vi "Begin.vi"(8 "error in":errorcluster) -> (0 "error out":errorcluster)   [LabVIEW 2014]
doc: "Called before other user functions, this VI is expected to open initial I/O refnums, load in file data, and do all program initialization. Notice that the <B>error out</B> terminal is simply used for data flow. Wiring it to other structures or subVIs ensures that this VI runs first."
uses:
  <vilib>/Rock Robotics/WPI/DriverStation/WPI_DriverStationRobotMode2.ctl
  <vilib>/Rock Robotics/WPI/Joystick/WPI_JoystickDeviceEnum.ctl
  <vilib>/Rock Robotics/WPI/Solenoid/WPI_SolenoidChannel.ctl
  <vilib>/Rock Robotics/SystemInterfaces/Typedef/FPGA_TypedefAnalogModuleForGyro.ctl
  <vilib>/Rock Robotics/SystemInterfaces/AI/FPGA_AIGyroChannel.ctl
  <vilib>/Rock Robotics/SystemInterfaces/AI/FPGA_AIChannel.ctl
  <vilib>/Rock Robotics/SystemInterfaces/Typedef/FPGA_TypedefAnalogModule.ctl
  <vilib>/Rock Robotics/WPI/Accelerometer/WPI_AccelerometerRange.ctl
  <vilib>/Rock Robotics/SystemInterfaces/DIO/FPGA_DIOChannel.ctl
  <vilib>/Rock Robotics/SystemInterfaces/Typedef/FPGA_TypedefDigitalModule.ctl
  <vilib>/Rock Robotics/WPI/CAN/TalonSRX/WPI_CANTalonSRX_APIControlMode.ctl
  Robot Global Data.vi
  <vilib>/Rock Robotics/WPI/Solenoid/WPI_SolenoidOpenSingle.vi
  <vilib>/Rock Robotics/WPI/Counter/WPI_CounterDigitalInputToDigitalSource.vi
  <vilib>/Rock Robotics/WPI/Accelerometer/InternalAccelerometer/WPI_AccelerometerInternalOpen.vi
  <vilib>/Rock Robotics/WPI/Switch/WPI_SwitchOpenLimit.vi
  <vilib>/Rock Robotics/WPI/RobotDrive/WPI_RobotDriveOpen4MotorWithCANTalonSRX.vi
  <vilib>/Rock Robotics/WPI/MotorControl/WPI_MotorControlOpenCANTalonSRX.vi
  <vilib>/Rock Robotics/WPI/Ultrasonic/WPI_SonarSRF04DigitalOpen.vi
  <vilib>/Rock Robotics/WPI/Ultrasonic/WPI_SonarSRF04DigitalRefNum Registry Set.vi
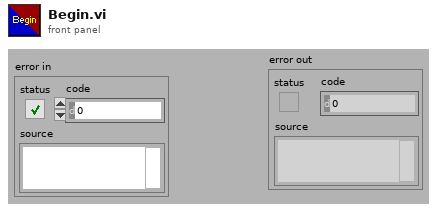
[diagram p1: front panel]
types:
  T1 = typedef "FPGA_DIOChannel.ctl" = enum8{"DIO 0", "DIO 1", "DIO 2", "DIO 3", "DIO 4", "DIO 5", "DIO 6", "DIO 7", "DIO 8", "DIO 9", "DIO MXP 0", "DIO MXP 1", "DIO MXP 2", "DIO MXP 3", "DIO MXP 4", "DIO MXP 5", "DIO MXP 6", "DIO MXP 7", "DIO MXP 8", "DIO MXP 9", "DIO MXP 10", "DIO MXP 11", "DIO MXP 12", "DIO MXP 13", "DIO MXP 14", "DIO MXP 15", "Invalid"}
  T2 = typedef "FPGA_TypedefDigitalModule.ctl" = enum16{"Controller 1"}
  T3 = typedef "WPI_CANTalonSRX_APIControlMode.ctl" = enum8{"Percent VBus", "Speed", "Position", "Slave", "Unchanged / Invalid"}
  T4 = typedef "WPI_AccelerometerRange.ctl" = enum16{"+/- 2 g", "+/- 4 g", "+/- 8 g"}
  T5 = typedef "FPGA_TypedefAnalogModule.ctl" = enum16{"Controller 1"}
  T6 = typedef "FPGA_AIChannel.ctl" = enum8{"AI 0", "AI 1", "AI 2", "AI 3", "AI MXP 0", "AI MXP 1", "AI MXP 2", "AI MXP 3", "Invalid"}
  T7 = typedef "FPGA_AIGyroChannel.ctl" = enum8{"AI 0", "AI 1", "Invalid"}
  T8 = typedef "FPGA_TypedefAnalogModuleForGyro.ctl" = enum16{"Controller 1"}
  T9 = typedef "WPI_SolenoidChannel.ctl" = enum8{"Solenoid 0", "Solenoid 1", "Solenoid 2", "Solenoid 3", "Solenoid 4", "Solenoid 5", "Solenoid 6", "Solenoid 7", "Invalid"}
  T10 = typedef "WPI_JoystickDeviceEnum.ctl" = enum16{"USB 0", "USB 1", "USB 2", "USB 3", "USB 4", "USB 5"}
  T11 = typedef "WPI_DriverStationRobotMode2.ctl" = enum16{"Autonomous Disabled", "Autonomous Enabled", "Teleop Disabled", "Teleop Enabled", "Disconnected", "Finish", "Test Disabled", "Test Enabled", "Emergency Stopped"}
  T12 = typedef "WPI_JoystickDevRef.ctl" = cluster{"Device":T10}
  T13 = typedef "WPI_DigitalInputDevRef.ctl" = cluster{"DevStatus":errorcluster, "DIO Channel":T1, "Controller":T2}
  T14 = typedef "WPI_AccelerometerDevRef.ctl" = cluster{"DevStatus":errorcluster, "Controller":T5, "Scaling":T15, "Analog Channels":T16, "I2C Bus":T17, "SPI Bus":T18, "Accel Range":T19, "ADXL345 Axes":T20, "Handle":i32, "Device Address":u8, "Accel Type":enum16{"Analog", "ADXL345 I2C", "ADXL345 SPI", "Internal"}}
  T15 = typedef "WPI_AccelerometerScaling.ctl" = cluster{"Gain (VoltsPerG)":dbl, "Center Voltage":dbl}
  T16 = typedef "WPI_AccelerometerAnalogChannels.ctl" = cluster{"X-Axis":T6, "Y-Axis":T6, "Z-Axis":T6}
  T17 = typedef "i2c_bus.ctl" = enum16{"I2C On-Board", "I2C MXP", "Invalid"}
  T18 = typedef "spi_bus.ctl" = enum16{"SPI On-Board, CS0", "SPI On-Board, CS1", "SPI On-Board, CS2", "SPI On-Board, CS3", "SPI MXP", "Invalid"}
  T19 = typedef "ADXL345 Range.ctl" = u8
  T20 = typedef "WPI_AccelerometerADXL345 Axes.ctl" = cluster{"X-Axis":bool, "Y-Axis":bool, "Z-Axis":bool}
  T21 = typedef "FPGA_CounterEncoderSourceConvertionLVSourceType.ctl" = cluster{"DevStatus":errorcluster, "AnalogTriggerMode?":bool, "DigitalMode":cluster{"Controller":T2, "DIO Channel":T22}, "AnalogTriggerMode":cluster{"AnalogTriggerIndex":T23, "OutputType":T24}}
  T22 = typedef "FPGA_DIODigitalSourceChannel.ctl" = enum8{"DIO 0", "DIO 1", "DIO 2", "DIO 3", "DIO 4", "DIO 5", "DIO 6", "DIO 7", "DIO 8", "DIO 9", "DIO MXP 0", "DIO MXP 1", "DIO MXP 2", "DIO MXP 3", "DIO MXP 4", "DIO MXP 5", "DIO MXP 6", "DIO MXP 7", "DIO MXP 8", "DIO MXP 9", "DIO MXP 10", "DIO MXP 11", "DIO MXP 12", "DIO MXP 13", "DIO MXP 14", "DIO MXP 15", "Disabled"}
  T23 = typedef "FPGA_AnalogTriggerIndex.ctl" = enum8{"Trig 0", "Trig 1", "Trig 2", "Trig 3", "Trig 4", "Trig 5", "Trig 6", "Trig 7", "Invalid"}
  T24 = typedef "FPGA_AnalogTriggerOutType.ctl" = enum16{"InWindow", "TriggerState", "Rising", "Falling"}
  T25 = typedef "WPI_RobotDriveDevRef.ctl" = cluster{"DevStatus":errorcluster, "Motors[]":T26[], "Square Inputs":bool, "Max Output":dbl}
  T26 = typedef "WPI_MotorControlDeviceRef.ctl" = cluster{"DeviceStatus":errorcluster, "Type":T27, "PWM":cluster{"Controller":T2, "PWM Channel":T28, "DeadBand":T29}, "CAN":cluster{"Device Number":u8, "Control Mode":T30, "Semaphore":T31, "Max Vout":dbl, "TalonSRX Control Mode":T3}, "Invert":bool, "TransformRef":T32, "InvTransformRef":T32}
  T27 = typedef "WPI_MotorControlType.ctl" = enum16{"PWM", "CAN", "CANTalonSRX"}
  T28 = typedef "FPGA_DIOPWMChannel.ctl" = enum8{"PWM 0", "PWM 1", "PWM 2", "PWM 3", "PWM 4", "PWM 5", "PWM 6", "PWM 7", "PWM 8", "PWM 9", "PWM MXP 0", "PWM MXP 1", "PWM MXP 2", "PWM MXP 3", "PWM MXP 4", "PWM MXP 5", "PWM MXP 6", "PWM MXP 7", "PWM MXP 8", "PWM MXP 9", "Invalid"}
  T29 = typedef "WPI_PWMDeadband.ctl" = cluster{"Name":string, "maxPositivePwm":i32, "minPositivePwm":i32, "centerPwm":i32, "maxNegativePwm":i32, "minNegativePwm":i32, "angularRange":u16}
  T30 = typedef "WPI_CANJaguar_ControlMode.ctl" = enum8{"Percent VBus", "Current", "Speed", "Position", "Voltage"}
  T31 = typedef "Semaphore RefNum" = refnum<k1>
  T32 = typedef "WPI_PWMTransform_ConPane.ctl" = refnum<vi>
  T33 = typedef "WPI_GyroDevRef.ctl" = cluster{"DevStatus":errorcluster, "Analog Module":T5, "Analog Channel":T6, "Offset":dbl, "Gain (VoltsPerDegree/Second)":dbl}
  T34 = typedef "WPI_EncoderDevRef.ctl" = cluster{"DevStatus":errorcluster, "EncoderIndex":T35, "CounterIndex":T36, "DistancePerCount":dbl, "Decoding Type":T37}
  T35 = typedef "FPGA_EncoderIdx.ctl" = enum8{"Enc 0", "Enc 1", "Enc 2", "Enc 3", "Enc 4", "Enc 5", "Enc 6", "Enc 7", "Invalid"}
  T36 = typedef "FPGA_CounterCtrSystemIndex.ctl" = enum8{"Ctr 0", "Ctr 1", "Ctr 2", "Ctr 3", "Ctr 4", "Ctr 5", "Ctr 6", "Ctr 7", "Invalid"}
  T37 = typedef "WPI_EncoderType.ctl" = enum16{"1x", "2x", "4x"}
  T38 = typedef "WPI_SolenoidDevRef.ctl" = cluster{"DevStatus":errorcluster, "Pneumatics Control Module":u8, "Forward Solenoid Channel":T9, "Reverse Solenoid Channel":T9}
  T39 = typedef "WPI_UltrasonicDeviceRef.ctl" = cluster{"DevStatus":errorcluster, "Ping Digital Controller":T2, "Echo Digital Controller":T2, "Ping Channel":T1, "Echo Channel":T1, "CntIndex":T36}
  T40 = typedef "WPI_PotentiometerDevRef.ctl" = cluster{"DevStatus":errorcluster, "Controller":T5, "Analog Channel":T6, "Invert Output":bool}
  T41 = typedef "WPI_SwitchDevRef.ctl" = cluster{"DevStatus":errorcluster, "DIO Channel":T1, "Controller":T2, "CntIndex":T36, "Normally Closed":bool}
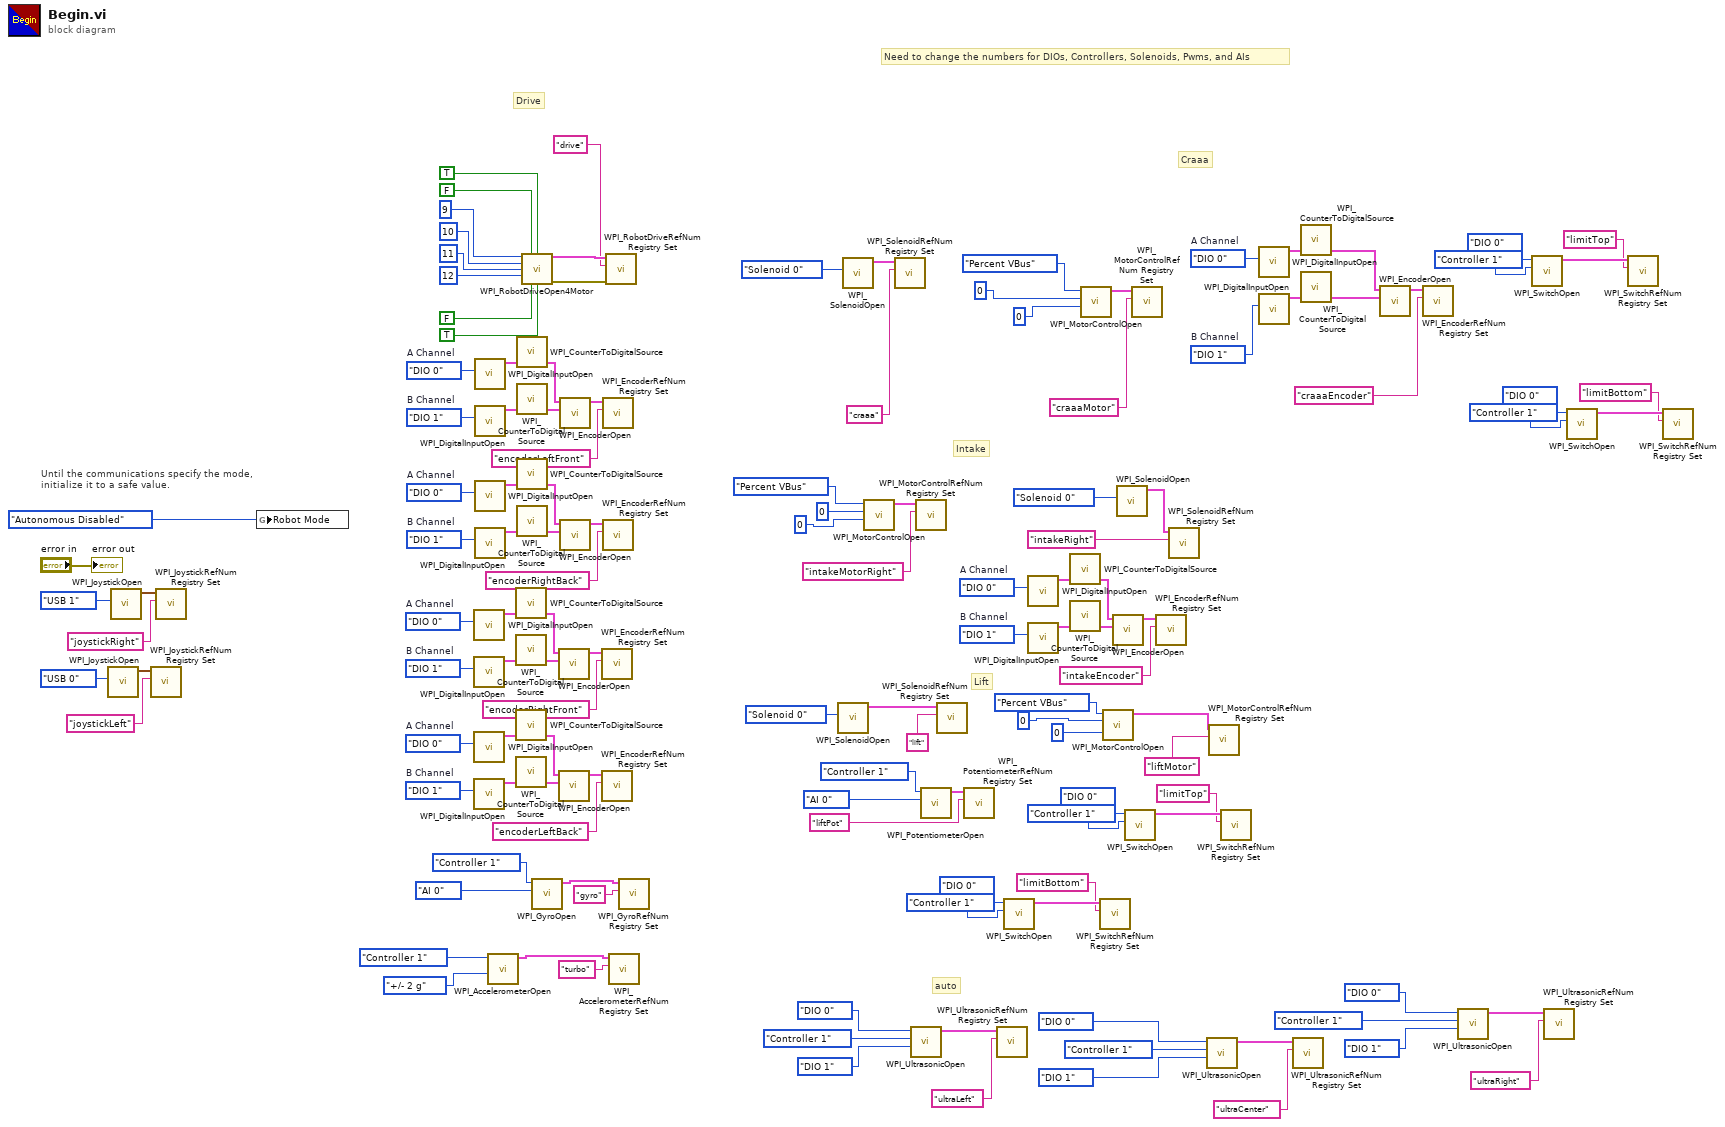
[diagram p0: block diagram]
diagram:
  w44 = FPGA_DIOChannel."DIO 1"  # B Channel
  w43 = FPGA_DIOChannel."DIO 0"  # A Channel
  w60 = FPGA_DIOChannel."DIO 1"  # B Channel
  w59 = FPGA_DIOChannel."DIO 0"  # A Channel
  w82 = FPGA_DIOChannel."DIO 1"  # B Channel
  w81 = FPGA_DIOChannel."DIO 0"  # A Channel
  w89 = FPGA_DIOChannel."DIO 1"  # B Channel
  w88 = FPGA_DIOChannel."DIO 0"  # A Channel
  w96 = FPGA_DIOChannel."DIO 1"  # B Channel
  w95 = FPGA_DIOChannel."DIO 0"  # A Channel
  w104 = FPGA_DIOChannel."DIO 1"  # B Channel
  w103 = FPGA_DIOChannel."DIO 0"  # A Channel
  # "auto"
  # "Need to change the numbers for DIOs, Controllers, Solenoids, Pwms, and AIs"
  # "Drive"
  # "Craaa"
  # "Intake"
  # "Lift"
  # "Until the communications specify the mode,\ninitialize it to a safe value."
  n1 = call <vilib>:"WPI_JoystickOpen.vi"("JoystickDevice"=WPI_JoystickDeviceEnum."USB 0") -> ("JoystickDevRef"=w129:T12)  [unwired: 10 in]
  n2 = call <vilib>:"WPI_JoystickOpen.vi"("JoystickDevice"=WPI_JoystickDeviceEnum."USB 1") -> ("JoystickDevRef"=w125:T12)  [unwired: 10 in]
  n3 = call <vilib>:"WPI_JoystickRefNum Registry Set.vi"("refnum name"="joystickLeft", "JoystickDevRef"=w129) -> ()  [unwired: 8 in, 2 out]
  n4 = call <vilib>:"WPI_JoystickRefNum Registry Set.vi"("refnum name"="joystickRight", "JoystickDevRef"=w125) -> ()  [unwired: 8 in, 2 out]
  n5 = global write "Robot Global Data.vi" "Robot Mode"(WPI_DriverStationRobotMode2."Autonomous Disabled" ("Robot Mode")) -> ()
  n6 = call <vilib>:"WPI_DigitalInputOpen.vi"("DIO Channel"=w95) -> ("DigitalInputDevRef"=w92:T13)  [unwired: 2 in, 8 out]
  n7 = call <vilib>:"WPI_DigitalInputOpen.vi"("DIO Channel"=w96) -> ("DigitalInputDevRef"=w93:T13)  [unwired: 2 in, 8 out]
  n8 = call <vilib>:"WPI_DigitalInputOpen.vi"("DIO Channel"=w81) -> ("DigitalInputDevRef"=w78:T13)  [unwired: 2 in, 8 out]
  n9 = call <vilib>:"WPI_DigitalInputOpen.vi"("DIO Channel"=w82) -> ("DigitalInputDevRef"=w79:T13)  [unwired: 2 in, 8 out]
  n10 = call <vilib>:"WPI_DigitalInputOpen.vi"("DIO Channel"=w103) -> ("DigitalInputDevRef"=w100:T13)  [unwired: 2 in, 8 out]
  n11 = call <vilib>:"WPI_DigitalInputOpen.vi"("DIO Channel"=w104) -> ("DigitalInputDevRef"=w101:T13)  [unwired: 2 in, 8 out]
  n12 = call <vilib>:"WPI_DigitalInputOpen.vi"("DIO Channel"=w88) -> ("DigitalInputDevRef"=w85:T13)  [unwired: 2 in, 8 out]
  n13 = call <vilib>:"WPI_DigitalInputOpen.vi"("DIO Channel"=w89) -> ("DigitalInputDevRef"=w86:T13)  [unwired: 2 in, 8 out]
  n14 = call-poly <vilib>:"WPI_AccelerometerOpen.vi"("Accel Range"=WPI_AccelerometerRange."+/- 2 g", "Controller"=FPGA_TypedefAnalogModule."Controller 1") -> ("AccelerometerDevRef"=w68:T14)  [unwired: 8 in, 1 out]
  n15 = call-poly <vilib>:"WPI_CounterToDigitalSource.vi"("DigitalInputDevRef"=w92) -> ("Digital Source"=w91:T21)  [unwired: 6 out]
  n16 = call-poly <vilib>:"WPI_CounterToDigitalSource.vi"("DigitalInputDevRef"=w93) -> ("Digital Source"=w94:T21)  [unwired: 6 out]
  n17 = call-poly <vilib>:"WPI_CounterToDigitalSource.vi"("DigitalInputDevRef"=w78) -> ("Digital Source"=w77:T21)  [unwired: 6 out]
  n18 = call-poly <vilib>:"WPI_CounterToDigitalSource.vi"("DigitalInputDevRef"=w79) -> ("Digital Source"=w80:T21)  [unwired: 6 out]
  n19 = call-poly <vilib>:"WPI_CounterToDigitalSource.vi"("DigitalInputDevRef"=w100) -> ("Digital Source"=w99:T21)  [unwired: 6 out]
  n20 = call-poly <vilib>:"WPI_CounterToDigitalSource.vi"("DigitalInputDevRef"=w101) -> ("Digital Source"=w102:T21)  [unwired: 6 out]
  n21 = call-poly <vilib>:"WPI_CounterToDigitalSource.vi"("DigitalInputDevRef"=w85) -> ("Digital Source"=w84:T21)  [unwired: 6 out]
  n22 = call-poly <vilib>:"WPI_CounterToDigitalSource.vi"("DigitalInputDevRef"=w86) -> ("Digital Source"=w87:T21)  [unwired: 6 out]
  n23 = call-poly <vilib>:"WPI_RobotDriveOpen4Motor.vi"("Rear Left Motor"=u8 9, "Rear Left Motor Inverted"=FALSE, "Rear Right Motor Inverted"=TRUE, "Rear Right Motor"=u8 10, "Front Left Motor"=u8 11, "Front Right Motor"=u8 12, "Front Left Motor Inverted"=FALSE, "Front Right Motor Inverted"=TRUE) -> ("RobotDriveDevRef"=w134:T25, "error out"=w132:errorcluster)  [unwired: 6 in]
  n24 = call <vilib>:"WPI_GyroOpen.vi"("Analog Channel"=FPGA_AIGyroChannel."AI 0", "Controller"=FPGA_TypedefAnalogModuleForGyro."Controller 1") -> ("GyroDevRef"=w98:T33)  [unwired: 7 in, 2 out]
  n25 = call <vilib>:"WPI_EncoderOpen.vi"("BSource"=w94, "ASource"=w91) -> ("EncoderDevRef"=w90:T34)  [unwired: 6 in, 3 out]
  n26 = call <vilib>:"WPI_EncoderOpen.vi"("BSource"=w80, "ASource"=w77) -> ("EncoderDevRef"=w76:T34)  [unwired: 6 in, 3 out]
  n27 = call <vilib>:"WPI_EncoderOpen.vi"("BSource"=w102, "ASource"=w99) -> ("EncoderDevRef"=w97:T34)  [unwired: 6 in, 3 out]
  n28 = call <vilib>:"WPI_EncoderOpen.vi"("BSource"=w87, "ASource"=w84) -> ("EncoderDevRef"=w83:T34)  [unwired: 6 in, 3 out]
  n29 = call <vilib>:"WPI_EncoderRefNum Registry Set.vi"("refnum name"="encoderRightFront", "EncoderDevRef"=w90) -> ()  [unwired: 8 in, 2 out]
  n30 = call <vilib>:"WPI_EncoderRefNum Registry Set.vi"("refnum name"="encoderLeftBack", "EncoderDevRef"=w76) -> ()  [unwired: 8 in, 2 out]
  n31 = call <vilib>:"WPI_EncoderRefNum Registry Set.vi"("refnum name"="encoderLeftFront", "EncoderDevRef"=w97) -> ()  [unwired: 8 in, 2 out]
  n32 = call <vilib>:"WPI_EncoderRefNum Registry Set.vi"("refnum name"="encoderRightBack", "EncoderDevRef"=w83) -> ()  [unwired: 8 in, 2 out]
  n33 = call <vilib>:"WPI_RobotDriveRefNum Registry Set.vi"("error in (no error)"=w132, "refnum name"="drive", "RobotDriveDevRef"=w134) -> ()  [unwired: 9 out]
  n34 = call <vilib>:"WPI_AccelerometerRefNum Registry Set.vi"("refnum name"="turbo", "AccelerometerDevRef"=w68) -> ()  [unwired: 8 in, 2 out]
  n35 = call <vilib>:"WPI_GyroRefNum Registry Set.vi"("refnum name"="gyro", "GyroDevRef"=w98) -> ()  [unwired: 8 in, 2 out]
  n36 = call-poly <vilib>:"WPI_SolenoidOpen.vi"("Solenoid Channel"=WPI_SolenoidChannel."Solenoid 0") -> ("SolenoidDevRef"=w117:T38)  [unwired: 9 in, 1 out]
  n37 = call-poly <vilib>:"WPI_SolenoidOpen.vi"("Solenoid Channel"=WPI_SolenoidChannel."Solenoid 0") -> ("SolenoidDevRef"=w119:T38)  [unwired: 9 in, 1 out]
  n38 = call-poly <vilib>:"WPI_MotorControlOpen.vi"("Master Device Number"=u8 0, "Device Number"=u8 0, "Control Mode"=WPI_CANTalonSRX_APIControlMode."Percent VBus") -> ("MotorControlDeviceRef"=w115:T26)  [unwired: 7 in, 1 out]
  n39 = call <vilib>:"WPI_SolenoidRefNum Registry Set.vi"("refnum name"="craaa", "SolenoidDevRef"=w119) -> ()  [unwired: 8 in, 2 out]
  n40 = call-poly <vilib>:"WPI_UltrasonicOpen.vi"("Echo DIO Channel"=FPGA_DIOChannel."DIO 1", "Echo Digital Controller"=FPGA_TypedefDigitalModule."Controller 1", "Ping DIO Channel"=FPGA_DIOChannel."DIO 0") -> ("SonarSRF04DevRef"=w28:T39)  [unwired: 7 in, 1 out]
  n41 = call <vilib>:"WPI_MotorControlRefNum Registry Set.vi"("refnum name"="intakeMotorRight", "MotorControlDevRef"=w115) -> ()  [unwired: 8 in, 2 out]
  n42 = call <vilib>:"WPI_PotentiometerOpen.vi"("Analog Channel"=FPGA_AIChannel."AI 0", "Controller"=FPGA_TypedefAnalogModule."Controller 1") -> ("PotDevRef"=w67:T40)  [unwired: 8 in, 1 out]
  n43 = call <vilib>:"WPI_SolenoidRefNum Registry Set.vi"("refnum name"="lift", "SolenoidDevRef"=w117) -> ()  [unwired: 8 in, 2 out]
  n44 = call <vilib>:"WPI_PotentiometerRefNum Registry Set.vi"("refnum name"="liftPot", "PotDevRef"=w67) -> ()  [unwired: 8 in, 2 out]
  n45 = call-poly <vilib>:"WPI_UltrasonicRefNum Registry Set.vi"("refnum name"="ultraLeft", "SonarSRF04DevRef"=w28) -> ()  [unwired: 8 in, 2 out]
  n46 = call-poly <vilib>:"WPI_SwitchOpen.vi"("DIO Channel"=FPGA_DIOChannel."DIO 0", "Controller"=FPGA_TypedefDigitalModule."Controller 1") -> ("SwitchDevRef"=w32:T41)  [unwired: 8 in, 1 out]
  n47 = call <vilib>:"WPI_DigitalInputOpen.vi"("DIO Channel"=w43) -> ("DigitalInputDevRef"=w40:T13)  [unwired: 2 in, 8 out]
  n48 = call <vilib>:"WPI_DigitalInputOpen.vi"("DIO Channel"=w44) -> ("DigitalInputDevRef"=w41:T13)  [unwired: 2 in, 8 out]
  n49 = call-poly <vilib>:"WPI_CounterToDigitalSource.vi"("DigitalInputDevRef"=w40) -> ("Digital Source"=w39:T21)  [unwired: 6 out]
  n50 = call-poly <vilib>:"WPI_CounterToDigitalSource.vi"("DigitalInputDevRef"=w41) -> ("Digital Source"=w42:T21)  [unwired: 6 out]
  n51 = call-poly <vilib>:"WPI_MotorControlOpen.vi"("Master Device Number"=u8 0, "Device Number"=u8 0, "Control Mode"=WPI_CANTalonSRX_APIControlMode."Percent VBus") -> ("MotorControlDeviceRef"=w116:T26)  [unwired: 7 in, 1 out]
  n52 = call <vilib>:"WPI_SwitchRefNum Registry Set.vi"("refnum name"="limitBottom", "SwitchDevRef"=w32) -> ()  [unwired: 8 in, 2 out]
  n53 = call-poly <vilib>:"WPI_MotorControlOpen.vi"("Master Device Number"=u8 0, "Device Number"=u8 0, "Control Mode"=WPI_CANTalonSRX_APIControlMode."Percent VBus") -> ("MotorControlDeviceRef"=w114:T26)  [unwired: 7 in, 1 out]
  n54 = call <vilib>:"WPI_EncoderOpen.vi"("BSource"=w42, "ASource"=w39) -> ("EncoderDevRef"=w38:T34)  [unwired: 6 in, 3 out]
  n55 = call-poly <vilib>:"WPI_SolenoidOpen.vi"("Solenoid Channel"=WPI_SolenoidChannel."Solenoid 0") -> ("SolenoidDevRef"=w118:T38)  [unwired: 9 in, 1 out]
  n56 = call-poly <vilib>:"WPI_SwitchOpen.vi"("DIO Channel"=FPGA_DIOChannel."DIO 0", "Controller"=FPGA_TypedefDigitalModule."Controller 1") -> ("SwitchDevRef"=w36:T41)  [unwired: 8 in, 1 out]
  n57 = call <vilib>:"WPI_MotorControlRefNum Registry Set.vi"("refnum name"="craaaMotor", "MotorControlDevRef"=w116) -> ()  [unwired: 8 in, 2 out]
  n58 = call <vilib>:"WPI_EncoderRefNum Registry Set.vi"("refnum name"="intakeEncoder", "EncoderDevRef"=w38) -> ()  [unwired: 8 in, 2 out]
  n59 = call <vilib>:"WPI_SolenoidRefNum Registry Set.vi"("refnum name"="intakeRight", "SolenoidDevRef"=w118) -> ()  [unwired: 8 in, 2 out]
  n60 = call-poly <vilib>:"WPI_UltrasonicOpen.vi"("Echo DIO Channel"=FPGA_DIOChannel."DIO 1", "Echo Digital Controller"=FPGA_TypedefDigitalModule."Controller 1", "Ping DIO Channel"=FPGA_DIOChannel."DIO 0") -> ("SonarSRF04DevRef"=w24:T39)  [unwired: 7 in, 1 out]
  n61 = call <vilib>:"WPI_MotorControlRefNum Registry Set.vi"("refnum name"="liftMotor", "MotorControlDevRef"=w114) -> ()  [unwired: 8 in, 2 out]
  n62 = call <vilib>:"WPI_SwitchRefNum Registry Set.vi"("refnum name"="limitTop", "SwitchDevRef"=w36) -> ()  [unwired: 8 in, 2 out]
  n63 = call <vilib>:"WPI_DigitalInputOpen.vi"("DIO Channel"=w59) -> ("DigitalInputDevRef"=w56:T13)  [unwired: 2 in, 8 out]
  n64 = call <vilib>:"WPI_DigitalInputOpen.vi"("DIO Channel"=w60) -> ("DigitalInputDevRef"=w57:T13)  [unwired: 2 in, 8 out]
  n65 = call-poly <vilib>:"WPI_UltrasonicRefNum Registry Set.vi"("refnum name"="ultraCenter", "SonarSRF04DevRef"=w24) -> ()  [unwired: 8 in, 2 out]
  n66 = call-poly <vilib>:"WPI_CounterToDigitalSource.vi"("DigitalInputDevRef"=w56) -> ("Digital Source"=w55:T21)  [unwired: 6 out]
  n67 = call-poly <vilib>:"WPI_CounterToDigitalSource.vi"("DigitalInputDevRef"=w57) -> ("Digital Source"=w58:T21)  [unwired: 6 out]
  n68 = call <vilib>:"WPI_EncoderOpen.vi"("BSource"=w58, "ASource"=w55) -> ("EncoderDevRef"=w54:T34)  [unwired: 6 in, 3 out]
  n69 = call <vilib>:"WPI_EncoderRefNum Registry Set.vi"("refnum name"="craaaEncoder", "EncoderDevRef"=w54) -> ()  [unwired: 8 in, 2 out]
  n70 = call-poly <vilib>:"WPI_UltrasonicOpen.vi"("Echo DIO Channel"=FPGA_DIOChannel."DIO 1", "Echo Digital Controller"=FPGA_TypedefDigitalModule."Controller 1", "Ping DIO Channel"=FPGA_DIOChannel."DIO 0") -> ("SonarSRF04DevRef"=w26:T39)  [unwired: 7 in, 1 out]
  n71 = call-poly <vilib>:"WPI_SwitchOpen.vi"("DIO Channel"=FPGA_DIOChannel."DIO 0", "Controller"=FPGA_TypedefDigitalModule."Controller 1") -> ("SwitchDevRef"=w52:T41)  [unwired: 8 in, 1 out]
  n72 = call-poly <vilib>:"WPI_UltrasonicRefNum Registry Set.vi"("refnum name"="ultraRight", "SonarSRF04DevRef"=w26) -> ()  [unwired: 8 in, 2 out]
  n73 = call-poly <vilib>:"WPI_SwitchOpen.vi"("DIO Channel"=FPGA_DIOChannel."DIO 0", "Controller"=FPGA_TypedefDigitalModule."Controller 1") -> ("SwitchDevRef"=w48:T41)  [unwired: 8 in, 1 out]
  n74 = call <vilib>:"WPI_SwitchRefNum Registry Set.vi"("refnum name"="limitTop", "SwitchDevRef"=w52) -> ()  [unwired: 8 in, 2 out]
  n75 = call <vilib>:"WPI_SwitchRefNum Registry Set.vi"("refnum name"="limitBottom", "SwitchDevRef"=w48) -> ()  [unwired: 8 in, 2 out]
  "error out" <- "error in"
